vi "DT_Triangle Manager_Del Boundary.vi"(9 "point idx":i32, 10 "triangle in":i32, 11 "Triangles In":i32[][](array[numeric])) -> (1 "adj triangle":i32, 2 "triangle out":i32, 3 "Triangles Out":i32[][](array[numeric]))   [LabVIEW 2017, in "NI_AAL_Geometry.lvlib"]
uses:
  <vilib>/Analysis/NI_AAL_Geometry.lvlib
  <vilib>/Analysis/geometry.llb/DT_Triangle Manager_Get Oppo Point_in Ghost.vi
  <vilib>/Analysis/geometry.llb/DT_Triangle Manager_Get Oppo Point.vi
  <vilib>/Analysis/geometry.llb/DT_Triangle Manager_Default Ghost Index.vi
  <vilib>/Analysis/geometry.llb/DT_Triangle Manager_Get Ghost Point.vi
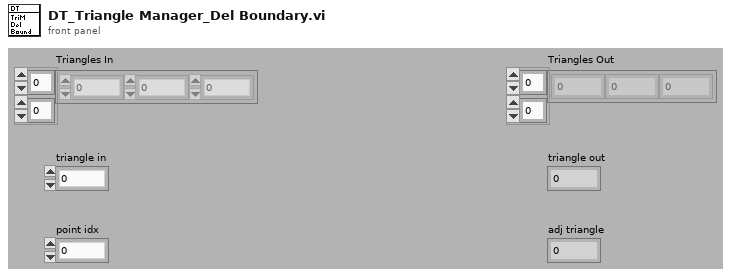
[diagram p1: front panel]
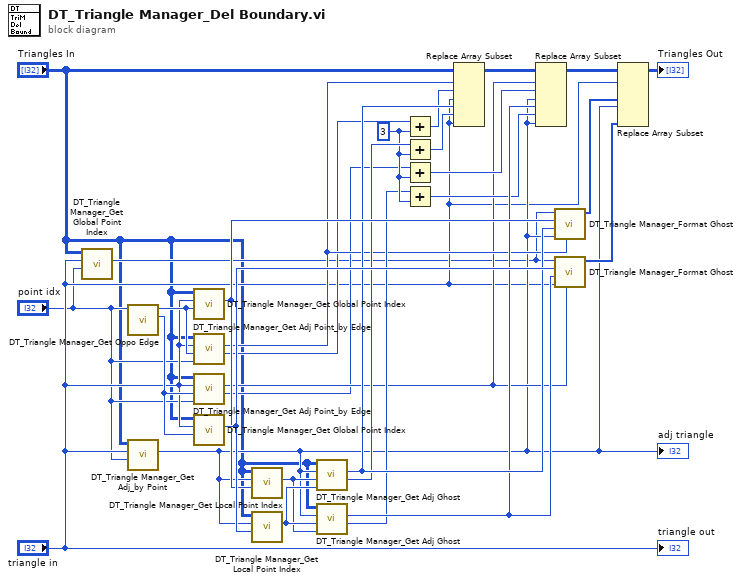
[diagram p0: block diagram]
diagram:
  w14 = 3 ("y")
  n1 = call <vilib>:"DT_Triangle Manager_Get Global Point Index.vi"("local idx"="point idx", "triangle"="triangle in", "Triangles"="Triangles In") -> ("global idx"=w3:i32)  [unwired: 8 out]
  n2 = call <vilib>:"DT_Triangle Manager_Get Oppo Edge.vi"("point idx"="point idx") -> ("oppo point idx 2"=w10:i32, "oppo point idx 1"=w11:i32)  [unwired: 9 out]
  n3 = call <vilib>:"DT_Triangle Manager_Get Adj_by Point.vi"("point idx"="point idx", "triangle"="triangle in", "Triangles In"="Triangles In") -> ("adj triangle"=w5:i32)  [unwired: 8 out]
  "adj triangle" <- w5
  n4 = call <vilib>:"DT_Triangle Manager_Get Global Point Index.vi"("local idx"=w11, "triangle"="triangle in", "Triangles"="Triangles In") -> ("global idx"=w25:i32)  [unwired: 8 out]
  n5 = call <vilib>:"DT_Triangle Manager_Get Adj Point_by Edge.vi"("point idx 2"="point idx", "point idx 1"=w11, "triangle"="triangle in", "Triangles In"="Triangles In") -> ("adj point idx"=w7:i32, "adj triangle"=w9:i32)  [unwired: 6 out]
  n6 = call <vilib>:"DT_Triangle Manager_Get Adj Point_by Edge.vi"("point idx 2"="point idx", "point idx 1"=w10, "triangle"="triangle in", "Triangles In"="Triangles In") -> ("adj point idx"=w6:i32, "adj triangle"=w8:i32)  [unwired: 6 out]
  n7 = call <vilib>:"DT_Triangle Manager_Get Global Point Index.vi"("local idx"=w10, "triangle"="triangle in", "Triangles"="Triangles In") -> ("global idx"=w26:i32)  [unwired: 8 out]
  n8 = call <vilib>:"DT_Triangle Manager_Get Local Point Index.vi"("global idx"=w25, "triangle"=w5, "Triangles"="Triangles In") -> ("local idx"=w23:i32)  [unwired: 8 out]
  n9 = call <vilib>:"DT_Triangle Manager_Get Local Point Index.vi"("global idx"=w26, "triangle"=w5, "Triangles"="Triangles In") -> ("local idx"=w24:i32)  [unwired: 8 out]
  n10 = call <vilib>:"DT_Triangle Manager_Get Adj Ghost.vi"("cur point idx"=w24, "cur base point idx"=w23, "cur triangle"=w5, "Triangles In"="Triangles In") -> ("next base point idx"=w17:i32, "next triangle"=w20:i32)  [unwired: 6 out]
  n11 = call <vilib>:"DT_Triangle Manager_Get Adj Ghost.vi"("cur point idx"=w23, "cur base point idx"=w24, "cur triangle"=w5, "Triangles In"="Triangles In") -> ("next base point idx"=w12:i32, "next triangle"=w18:i32)  [unwired: 6 out]
  n12 = Add(x=w7, y=w14) -> (x+y=w16:i32)
  n13 = Add(x=w17, y=w14) -> (x+y=w19:i32)
  n14 = Add(x=w6, y=w14) -> (x+y=w15:i32)
  n15 = Add(x=w12, y=w14) -> (x+y=w13:i32)
  n16 = Replace Array Subset(array="Triangles In", new element #1="triangle in", index (row) #1=w9, index (col) #1=w16, new element #2="triangle in", index (row) #2=w20, index (col) #2=w19) -> (w22:i32[][])
  n17 = Replace Array Subset(array=w22, new element #1=w5, index (row) #1=w8, index (col) #1=w15, new element #2=w5, index (row) #2=w18, index (col) #2=w13) -> (w21:i32[][])
  n18 = call <vilib>:"DT_Triangle Manager_Format Ghost.vi"("triangle"=w9, "p 2 triangle"=w5, "p 1 triangle"=w20, "p 2"=w25, "p 1"=w3) -> ("Triangle"=w28:i32[])  [unwired: 6 out]
  n19 = call <vilib>:"DT_Triangle Manager_Format Ghost.vi"("triangle"=w8, "p 2 triangle"="triangle in", "p 1 triangle"=w18, "p 2"=w26, "p 1"=w3) -> ("Triangle"=w27:i32[])  [unwired: 6 out]
  n20 = Replace Array Subset(array=w21, new element #1=w28, index (row) #1="triangle in", new element #2=w27, index (row) #2=w5) -> (→"Triangles Out":i32[][])  [unwired: 2 in]
  "triangle out" <- "triangle in"
